vi "GEOM_API.vi"(7 "Cmd":string, 11 "error in":errorcluster) -> (4 "ImmedReplyString":string, 15 "error out":errorcluster)   [LabVIEW 2016]
uses:
  private/vis/GEOM_Coords.ctl
  private/vis/GEOM_VAR_action.ctl
  DBSHAND/private/vis/DatabaseHand_Element_Set(bool).vi
  DBSHAND/private/vis/DatabaseHand_Element_Set(string).vi
  DBSHAND/private/vis/DatabaseHand_Element_Get(bool).vi
panel:
  in  "optimize":bool=TRUE
  in  "overwcs":path
  in  "hdrmoddir":path
  out "header template":path
  out "ConfigFile":path
  in  "bin_correction_type":string="add2pre"
  out "FPA":string
  in  "correction_type":string="simetrical_used_columns"
  in  "ConfigVariables":string[][](table)=[["DATABASE", "path", "GEOM_API.vi", "database_path", "/home/ArcVIEW/Modules/GEOM/public/database", "PATH"], ["ROI", "correction", "GEOM_API.vi", "correction_type", "simetrical_used_columns", "STR"], ["BINNING", "correction", "GEOM_API.vi", "bin_correction_type", "add2pre", "STR"], ["HDRINFO", "hdrmoddir", "GEOM_API.vi", "hdrmoddir", "", "PATH"], ["HDRINFO", "overwcs", "GEOM_API.vi", "overwcs", "", "PATH"], ["MISC", "optimize", "GEOM_API.vi", "optimize", "", "BOOL"]]
  out "Initialized":bool
  in  "database_path":path=path "/__none__"
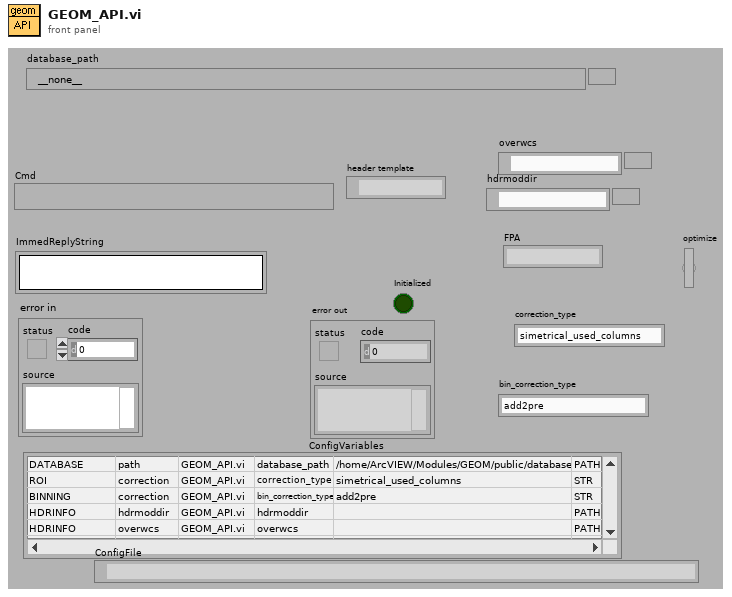
[diagram p1: front panel]
types:
  T1 = typedef "GEOM_VAR_action.ctl" = enum16{"read", "write"}
  T2 = typedef "GEOM_Coords.ctl" = cluster{"xstart":u32, "ystart":u32, "xsize":u32, "ysize":u32}
  T3 = typedef "DatabaseHand_RefNum.ctl" = refnum<vi>
  T4 = typedef "GEOM_HeaderModule.ctl" = cluster{"name":string, "Keys":string[][]}
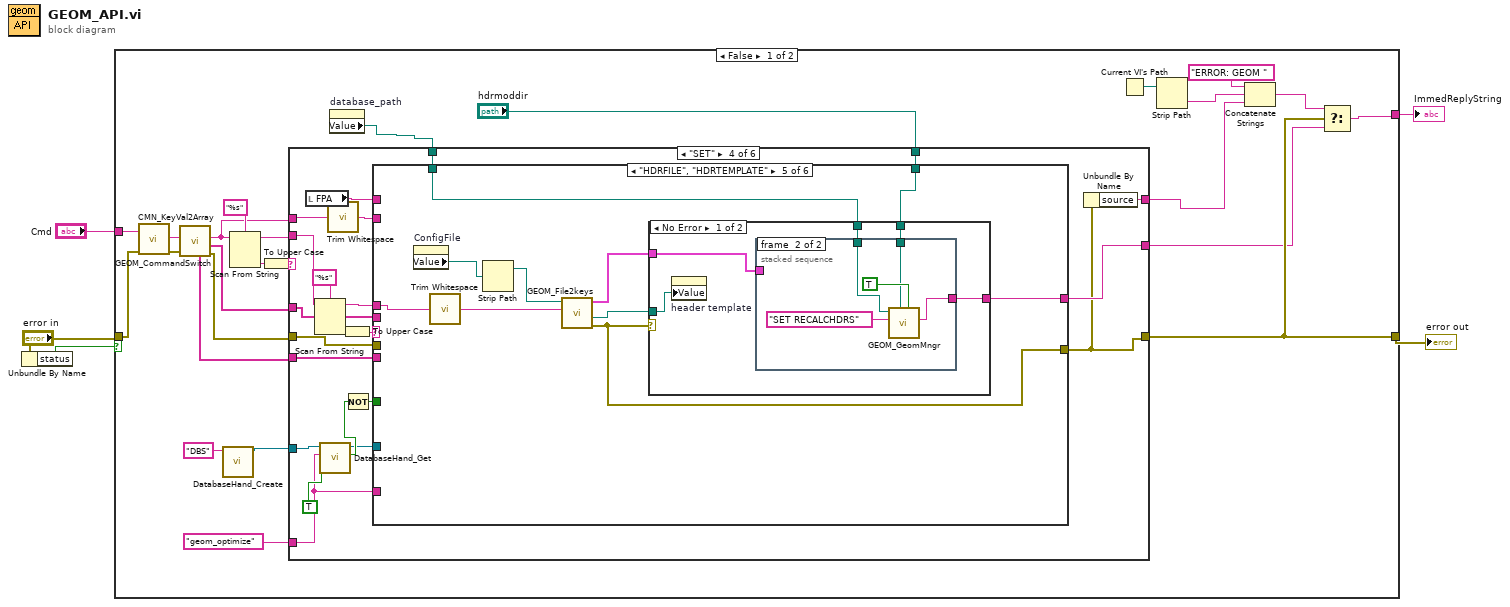
[diagram p0: block diagram]
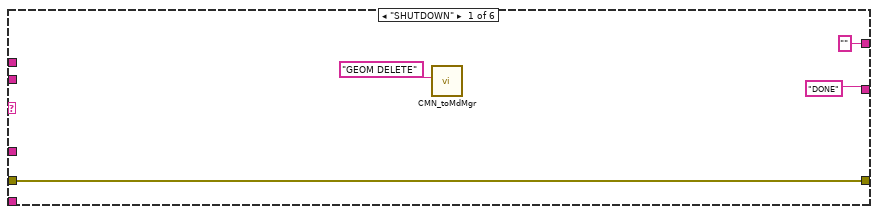
[diagram p2: hidden frame]
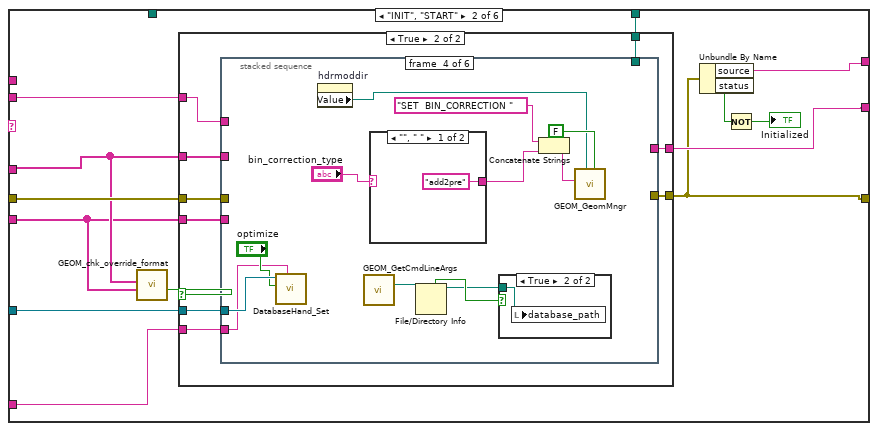
[diagram p3: hidden frame]
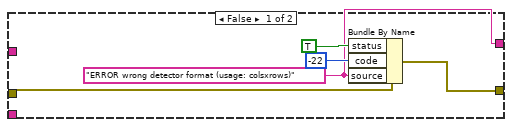
[diagram p4: hidden frame]
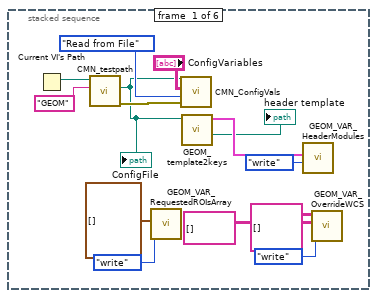
[diagram p5: hidden frame]
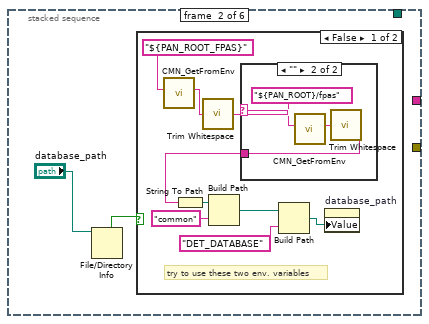
[diagram p6: hidden frame]
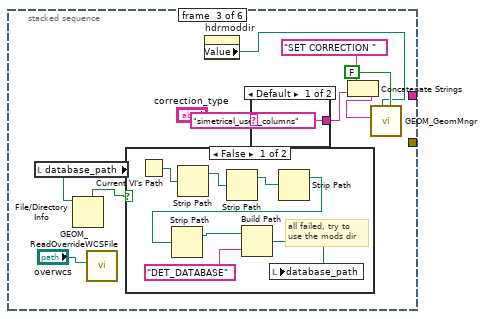
[diagram p9: hidden frame]
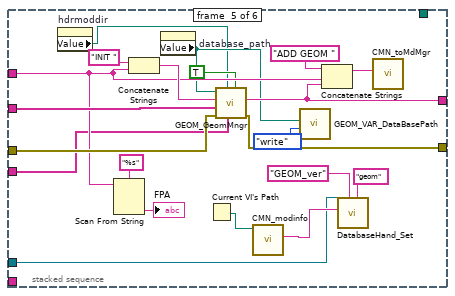
[diagram p14: hidden frame]
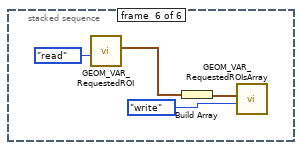
[diagram p15: hidden frame]
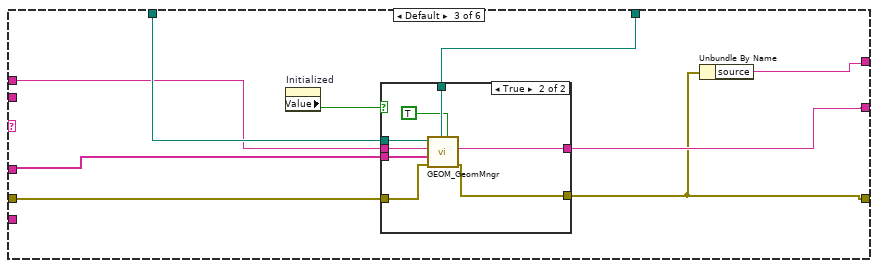
[diagram p16: hidden frame]
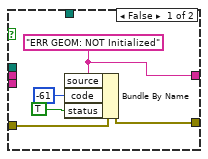
[diagram p17: hidden frame]
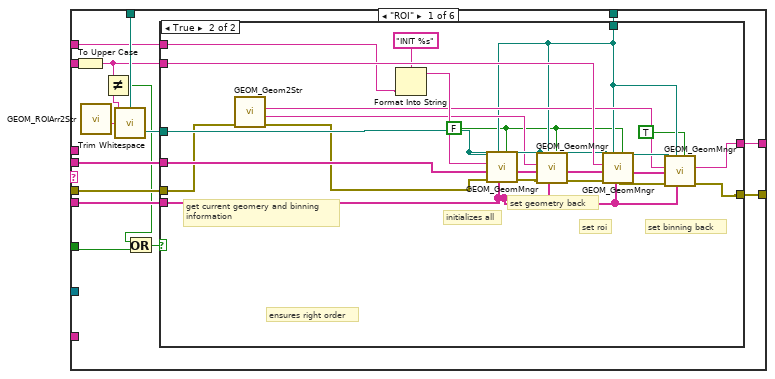
[diagram p18: hidden frame]
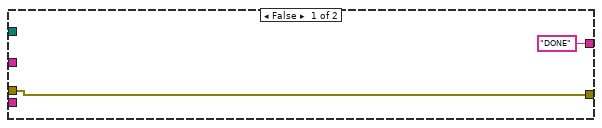
[diagram p19: hidden frame]
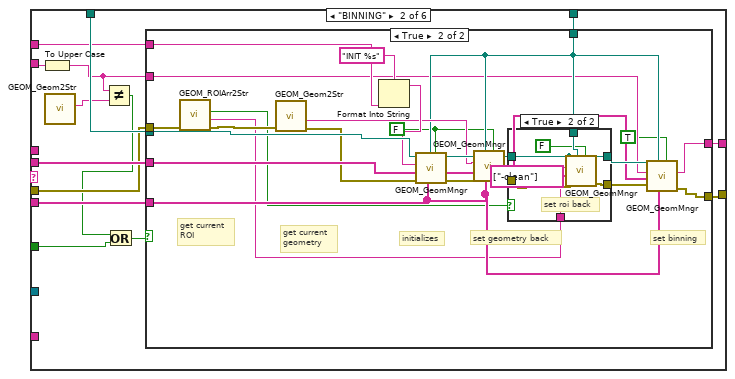
[diagram p20: hidden frame]
diagram:
  n1 = Unbundle By Name("error in") -> ("status"=w3:bool)
  n2 = case shown="False" w3 {
    tunnel: "error in" -> [w17 w457]
    tunnel: [w30 w457] -> w1
    tunnel: [w29 ""] -> w5
    tunnel: "Cmd" -> [w18 _]
    frame False {
      n3 = call "CMN_KeyVal2Array.vi"("error in (no error)"=w17, "command in"=w18) -> ("error out"=w16:errorcluster, "commands out"=w12:string)  [unwired: 1 in, 6 out]
      n4 = call "GEOM_CommandSwitch.vi"("error in (no error)"=w16, "command in"=w12) -> ("error out"=w15:errorcluster, "swhitches"=w13:string[], "command out"=w14:string, "arguments"=w11:string[])  [unwired: 6 out]
      n5 = call "DatabaseHand_Create.vi"("Name"="DBS") -> ("Database RefNum out"=w8:T3)  [unwired: 1 in, 9 out]
      n6 = Scan From String(format string="%s" ("Format String"), input string=w14) -> (remaining string=w20:string, output 1=w28:string)  [unwired: 2 in, 3 out]
      n7 = To Upper Case(1:w28) -> (0:w19:string)
      n8 = property on="database_path" class="Path"() -> ("Value"=w6:path)  [unwired: 2 in, 2 out]
      n9 = case shown="\"SET\"" w19 {
        tunnel: w15 -> [w32 w47 w157 w188 w405 w450]
        tunnel: [w32 w45 w155 w184 w403 w449] -> w30
        tunnel: ["" ("source") w44 w154 w183 w402 w448] -> w22
        tunnel: ["DONE" w46 w156 w185 w404 w448] -> w21
        tunnel: w20 -> [_ w43 _ w192 w398 _]
        tunnel: w14 -> [_ _ w151 w189 w399 _]
        tunnel: w6 -> [_ _ w153 w186 w401 _]
        tunnel: w13 -> [_ w40 w152 w187 w400 w455]
        tunnel: w11 -> [_ w39 _ w181 _ _]
        tunnel: "hdrmoddir" -> [_ w37 w149 w180 w393 _]
        tunnel: w8 -> [_ w36 _ w176 w392 _]
        tunnel: "geom_optimize" ("name") -> [_ w35 _ w171 w391 _]
        frame "SHUTDOWN" {
          n10 = call "CMN_toMdMgr.vi"("command"="GEOM DELETE" ("Command")) -> ()  [unwired: 10 out]
        }
        frame "INIT", "START" {
          n11 = call "GEOM_chk_override_format.vi"("arguments"=w39, "switches"=w40) -> ("format OK"=w38:bool)  [unwired: 9 out]
          n12 = case shown="True" w38 {
            tunnel: w47 -> [w52 w61]
            tunnel: [w48 w60] -> w46
            tunnel: [w49 w59] -> w45
            tunnel: w43 -> [_ w58]
            tunnel: w40 -> [_ w57]
            tunnel: w39 -> [_ w56]
            tunnel: w37 -> [_ w55]
            tunnel: w36 -> [_ w54]
            tunnel: w35 -> [_ w53]
            frame False {
              w48 = "ERROR wrong detector format (usage: colsxrows)" ("source")
              n13 = Bundle By Name(cluster=w52, "status"=TRUE, "code"=-22, "source"=w48) -> (w49:errorcluster)
            }
            frame True {
              n14 = stacked-sequence {
                tunnel: w61 -> [_ _ _ _ w144 _]
                tunnel: [_ _ _ _ w137 _] -> w60
                tunnel: [_ _ _ _ w143 _] -> w59
                tunnel: w58 -> [_ _ _ _ w136 _]
                tunnel: w57 -> [_ _ _ _ w140 _]
                tunnel: w56 -> [_ _ _ _ w129 _]
                tunnel: w55 -> [_ _ _ _ _ _]
                tunnel: w54 -> [_ _ _ w113 w125 _]
                tunnel: w53 -> [_ _ _ w111 _ _]
                frame #0 {
                  n15 = Current VI's Path() -> (path=w75:path)
                  n16 = call "CMN_testpath.vi"("ModuleName"="GEOM", "caller Path"=w75) -> ("error out"=w72:errorcluster, "ConfigFile"=w70:path)  [unwired: 1 in, 7 out]
                  "ConfigFile" <- w70
                  n17 = call "GEOM_VAR_RequestedROIsArray.vi"("Action"=GEOM_VAR_action."write", "ROIs"=T2[] []) -> ()  [unwired: 10 out]
                  n18 = call "CMN_ConfigVals.vi"("error in (no error)"=w72, "Action"=enum16{"Read from File", "Write to File"}."Read from File", "ConfigVariables"="ConfigVariables", "configuration file path"=w70) -> ()  [unwired: 8 out]
                  n19 = call "GEOM_template2keys.vi"("file"=w70) -> ("header template"=→"header template":path, "HeaderModules"=w69:T4[])  [unwired: 1 in, 8 out]
                  n20 = call "GEOM_VAR_HeaderModules.vi"("Action"=GEOM_VAR_action."write", "GEOM_HeaderModules"=w69) -> ()  [unwired: 10 out]
                  n21 = call "GEOM_VAR_OverrideWCS.vi"("Action"=GEOM_VAR_action."write", "override headers"=string[][] [], "override headers mext"=string[][][] []) -> ()  [unwired: 9 out]
                }
                frame #1 {
                  n22 = File/Directory Info(path="database_path") -> (directory=w77:bool)  [unwired: 1 in, 6 out]
                  n23 = case shown="False" w77 {
                    frame False {
                      # "try to use these two env. variables"
                      n24 = call "CMN_GetFromEnv.vi"("str in"="${PAN_ROOT_FPAS}") -> ("str out"=w85:string)  [unwired: 10 out]
                      n25 = call <vilib>:"Trim Whitespace.vi"("string"=w85) -> ("trimmed string"=w84:string)  [unwired: 1 in]
                      n26 = case shown="\"\"" w84 {
                        selector: w84 -> [w87 _]
                        tunnel: [w87 w88] -> w83
                        frame Default {
                        }
                        frame "" {
                          n27 = call "CMN_GetFromEnv.vi"("str in"="${PAN_ROOT}/fpas") -> ("str out"=w89:string)  [unwired: 10 out]
                          n28 = call <vilib>:"Trim Whitespace.vi"("string"=w89) -> ("trimmed string"=w88:string)  [unwired: 1 in]
                        }
                      }
                      n29 = String To Path(string=w83) -> (path=w82:path)
                      n30 = Build Path(base path=w82, name or relative path="common") -> (appended path=w80:path)
                      n31 = Build Path(base path=w80, name or relative path="DET_DATABASE") -> (appended path=w78:path)
                      n32 = property on="database_path" class="Path"("Value"=w78) -> ()  [unwired: 2 in, 2 out]
                    }
                    frame True {
                      # "specified in config file"
                    }
                  }
                }
                frame #2 {
                  n33 = local read "database_path"() -> (w99:path)
                  n34 = File/Directory Info(path=w99) -> (directory=w98:bool)  [unwired: 1 in, 6 out]
                  n35 = call "GEOM_ReadOverrideWCSFile.vi"("Path"="overwcs") -> ()  [unwired: 11 out]
                  n36 = case shown="False" w98 {
                    frame False {
                      # "all failed, try to\nuse the mods dir"
                      n37 = Current VI's Path() -> (path=w108:path)
                      n38 = Strip Path(path=w108) -> (stripped path=w107:path)  [unwired: 1 out]
                      n39 = Strip Path(path=w107) -> (stripped path=w106:path)  [unwired: 1 out]
                      n40 = Strip Path(path=w106) -> (stripped path=w105:path)  [unwired: 1 out]
                      n41 = Strip Path(path=w105) -> (stripped path=w104:path)  [unwired: 1 out]
                      n42 = Build Path(base path=w104, name or relative path="DET_DATABASE") -> (appended path=w102:path)
                      n43 = local write "database_path"(w102) -> ()
                    }
                    frame True {
                    }
                  }
                  n44 = property on="hdrmoddir" class="Path"() -> ("Value"=w91:path)  [unwired: 2 in, 2 out]
                  n45 = case shown="Default" "correction_type" {
                    selector: "correction_type" -> [_ w101]
                    tunnel: ["simetrical_used_columns" w101] -> w95
                    frame Default {
                    }
                    frame "simetrical_all_columns" {
                    }
                  }
                  n46 = Concatenate Strings("SET CORRECTION " ("string"), w95) -> (w94:string)
                  n47 = call "GEOM_GeomMngr.vi"("calc headers?"=FALSE, "hdrmodspath"=w91, "command"=w94) -> ()  [unwired: 4 in, 5 out]
                }
                frame #3 {
                  n48 = call-poly "DatabaseHand_Set.vi"("name"=w111, "value"="optimize", "Database RefNum in"=w113) -> ()  [unwired: 5 in, 4 out]
                  n49 = property on="hdrmoddir" class="Path"() -> ("Value"=w109:path)  [unwired: 2 in, 2 out]
                  n50 = call "GEOM_GetCmdLineArgs.vi"() -> ("det_database"=w116:path)  [unwired: 15 out]
                  n51 = case shown="\"\", \" \"" "bin_correction_type" {
                    selector: "bin_correction_type" -> [_ w123]
                    tunnel: ["add2pre" w123] -> w117
                    frame "", " " {
                    }
                    frame Default {
                    }
                  }
                  n52 = File/Directory Info(path=w116) -> (path out=w114:path, directory=w115:bool)  [unwired: 1 in, 5 out]
                  n53 = case shown="True" w115 {
                    tunnel: w114 -> [_ w121]
                    frame False {
                    }
                    frame True {
                      n54 = local write "database_path"(w121) -> ()
                    }
                  }
                  n55 = Concatenate Strings("SET  BIN_CORRECTION " ("string"), w117) -> (w118:string)
                  n56 = call "GEOM_GeomMngr.vi"("calc headers?"=FALSE, "hdrmodspath"=w109, "command"=w118) -> ()  [unwired: 4 in, 5 out]
                }
                frame #4 {
                  n57 = property on="hdrmoddir" class="Path"() -> ("Value"=w124:path)  [unwired: 2 in, 2 out]
                  n58 = Scan From String(format string="%s", input string=w136) -> (output 1=→"FPA":string)  [unwired: 2 in, 4 out]
                  n59 = Concatenate Strings("INIT ", w136) -> (w141:string)
                  n60 = property on="database_path" class="Path"() -> ("Value"=w127:path)  [unwired: 2 in, 2 out]
                  n61 = Current VI's Path() -> (path=w133:path)
                  n62 = call "GEOM_GeomMngr.vi"("calc headers?"=TRUE, "arguments"=w129, "hdrmodspath"=w124, "error in (no error)"=w144, "switches"=w140, "command"=w141, "database path"=w127) -> ("error out"=w143:errorcluster, "response"=w137:string)  [unwired: 3 out]
                  n63 = call "CMN_modinfo.vi"("caller path"=w133) -> ("INFO"=w132:string)  [unwired: 2 in, 8 out]
                  n64 = call "GEOM_VAR_DataBasePath.vi"("Action"=GEOM_VAR_action."write", "Path"=w127) -> ()  [unwired: 10 out]
                  n65 = Concatenate Strings("ADD GEOM " ("command"), w136, w137) -> (w138:string)
                  n66 = call-poly "DatabaseHand_Set.vi"("group"="geom", "name"="GEOM_ver", "value"=w132, "Database RefNum in"=w125) -> ()  [unwired: 4 in, 4 out]
                  n67 = call "CMN_toMdMgr.vi"("command"=w138) -> ()  [unwired: 10 out]
                }
                frame #5 {
                  n68 = call "GEOM_VAR_RequestedROI.vi"("Action"=GEOM_VAR_action."read") -> ("GEOM_RequestedROI out"=w145:T2)  [unwired: 1 in, 9 out]
                  n69 = Build Array(w145) -> (w147:T2[])
                  n70 = call "GEOM_VAR_RequestedROIsArray.vi"("Action"=GEOM_VAR_action."write", "ROIs"=w147) -> ()  [unwired: 10 out]
                }
              }
            }
          }
          n71 = Unbundle By Name(w45) -> ("source"=w44:string, "status"=w42:bool)
          n72 = Not(x=w42) -> (.not. x?=→"Initialized":bool)
        }
        frame Default {
          n73 = property on="Initialized" class="Bool (strict)"() -> ("Value"=w150:bool)  [unwired: 2 in, 2 out]
          n74 = case shown="True" w150 {
            tunnel: w157 -> [w162 w170]
            tunnel: [w159 w169] -> w156
            tunnel: [w161 w168] -> w155
            tunnel: w153 -> [_ w167]
            tunnel: w152 -> [_ w166]
            tunnel: w151 -> [_ w165]
            tunnel: w149 -> [_ w164]
            frame False {
              w159 = "ERR GEOM: NOT Initialized" ("source")
              n75 = Bundle By Name(cluster=w162, "source"=w159, "code"=-61, "status"=TRUE) -> (w161:errorcluster)
            }
            frame True {
              n76 = call "GEOM_GeomMngr.vi"("calc headers?"=TRUE, "hdrmodspath"=w164, "error in (no error)"=w170, "switches"=w166, "command"=w165, "database path"=w167) -> ("error out"=w168:errorcluster, "response"=w169:string)  [unwired: 1 in, 3 out]
            }
          }
          n77 = Unbundle By Name(w155) -> ("source"=w154:string)
        }
        frame "SET" {
          n78 = local read "FPA"() -> (w182:string)
          n79 = Scan From String(format string="%s", input string=w192) -> (remaining string=w177:string, output 1=w191:string)  [unwired: 2 in, 3 out]
          n80 = call-poly "DatabaseHand_Get.vi"("default value"=TRUE, "name"=w171, "Database RefNum in"=w176) -> ("value"=w174:bool, "Database RefNum out"=w172:T3)  [unwired: 2 in, 5 out]
          n81 = call <vilib>:"Trim Whitespace.vi"("string"=w189) -> ("trimmed string"=w179:string)  [unwired: 1 in]
          n82 = To Upper Case(1:w191) -> (0:w178:string)
          n83 = Not(x=w174) -> (.not. x?=w173:bool)
          n84 = case shown="\"HDRFILE\", \"HDRTEMPLATE\"" w178 {
            tunnel: w179 -> [w207 w234 w282 _ _ w375]
            tunnel: w188 -> [w201 w235 w283 _ _ w374]
            tunnel: w187 -> [w202 w238 w285 _ _ w373]
            tunnel: w186 -> [w206 w242 w287 _ w342 w372]
            tunnel: [w205 w241 w290 errorcluster {"status"=FALSE, "code"=0, "source"=""} ("error out") w347 w371] -> w184
            tunnel: [w204 w240 w289 w327 w346 w370] -> w185
            tunnel: w182 -> [w203 w239 w288 _ _ _]
            tunnel: w181 -> [w200 w237 w284 _ _ w369]
            tunnel: w180 -> [w199 w236 w286 _ w343 w368]
            tunnel: w177 -> [_ _ _ w330 w349 _]
            tunnel: w173 -> [w195 w230 w276 _ _ _]
            tunnel: w172 -> [_ _ _ w332 _ _]
            tunnel: w171 -> [_ _ _ w331 _ _]
            frame "ROI" {
              n85 = To Upper Case(1:w207) -> (0:w198:string)
              n86 = call "GEOM_ROIArr2Str.vi"() -> ("ROI command"=w197:string)  [unwired: 1 in, 10 out]
              n87 = call <vilib>:"Trim Whitespace.vi"("string"=w197) -> ("trimmed string"=w196:string)  [unwired: 1 in]
              n88 = Not Equal?(x=w198, y=w196) -> (x != y?=w194:bool)
              n89 = Or(x=w194, y=w195) -> (x .or. y?=w193:bool)
              n90 = case shown="True" w193 {
                tunnel: w198 -> [_ w228]
                tunnel: w206 -> [_ w226]
                tunnel: [w209 w225] -> w205
                tunnel: ["DONE" ("response") w224] -> w204
                tunnel: w203 -> [_ w222]
                tunnel: w202 -> [_ w216]
                tunnel: w201 -> [w209 w215]
                tunnel: w200 -> [_ w213]
                tunnel: w199 -> [_ w212]
                frame False {
                }
                frame True {
                  w211 = FALSE ("calc headers?")
                  # "get current geomery and binning\ninformation"
                  # "ensures right order"
                  # "set binning back"
                  # "set roi"
                  # "set geometry back"
                  # "initializes all"
                  n91 = call "GEOM_Geom2Str.vi"("error in (no error)"=w215) -> ("error out"=w214:errorcluster, "geometry command"=w217:string, "binning command"=w220:string)  [unwired: 8 out]
                  n92 = Format Into String(format string="INIT %s", w222) -> (resulting string=w221:string)  [unwired: 2 in, 1 out]
                  n93 = call "GEOM_GeomMngr.vi"("calc headers?"=w211, "arguments"=w213, "hdrmodspath"=w212, "error in (no error)"=w214, "switches"=w216, "command"=w221, "database path"=w226) -> ("error out"=w219:errorcluster)  [unwired: 4 out]
                  n94 = call "GEOM_GeomMngr.vi"("calc headers?"=w211, "arguments"=w213, "hdrmodspath"=w212, "error in (no error)"=w219, "switches"=w216, "command"=w217, "database path"=w226) -> ("error out"=w218:errorcluster)  [unwired: 4 out]
                  n95 = call "GEOM_GeomMngr.vi"("calc headers?"=w211, "arguments"=w213, "hdrmodspath"=w212, "error in (no error)"=w218, "switches"=w216, "command"=w228, "database path"=w226) -> ("error out"=w227:errorcluster)  [unwired: 4 out]
                  n96 = call "GEOM_GeomMngr.vi"("calc headers?"=TRUE, "arguments"=w213, "hdrmodspath"=w212, "error in (no error)"=w227, "switches"=w216, "command"=w220, "database path"=w226) -> ("error out"=w225:errorcluster, "response"=w224:string)  [unwired: 3 out]
                }
              }
            }
            frame "BINNING" {
              n97 = To Upper Case(1:w234) -> (0:w233:string)
              n98 = call "GEOM_Geom2Str.vi"() -> ("binning command"=w232:string)  [unwired: 1 in, 10 out]
              n99 = Not Equal?(x=w233, y=w232) -> (x != y?=w231:bool)
              n100 = Or(x=w231, y=w230) -> (x .or. y?=w229:bool)
              n101 = case shown="True" w229 {
                tunnel: w242 -> [_ w266]
                tunnel: [w244 w262] -> w241
                tunnel: ["DONE" ("response") w260] -> w240
                tunnel: w239 -> [_ w259]
                tunnel: w238 -> [_ w257]
                tunnel: w237 -> [_ w253]
                tunnel: w236 -> [_ w252]
                tunnel: w235 -> [w244 w251]
                tunnel: w233 -> [_ w247]
                frame False {
                  # "nothing to do"
                }
                frame True {
                  w246 = FALSE ("calc headers?")
                  # "set binning"
                  # "set geometry back"
                  # "initializes"
                  # "get current \ngeometry"
                  # "get current \nROI"
                  n102 = call "GEOM_ROIArr2Str.vi"("error in (no error)"=w251) -> ("error out"=w250:errorcluster, "ROI command"=w248:string, "defined?"=w249:bool)  [unwired: 8 out]
                  n103 = call "GEOM_Geom2Str.vi"("error in (no error)"=w250) -> ("error out"=w254:errorcluster, "geometry command"=w255:string)  [unwired: 9 out]
                  n104 = Format Into String(format string="INIT %s", w259) -> (resulting string=w264:string)  [unwired: 2 in, 1 out]
                  n105 = call "GEOM_GeomMngr.vi"("calc headers?"=w246, "arguments"=w253, "hdrmodspath"=w252, "error in (no error)"=w254, "switches"=w257, "command"=w264, "database path"=w266) -> ("error out"=w258:errorcluster)  [unwired: 4 out]
                  n106 = call "GEOM_GeomMngr.vi"("calc headers?"=w246, "arguments"=w253, "hdrmodspath"=w252, "error in (no error)"=w258, "switches"=w257, "command"=w255, "database path"=w266) -> ("error out"=w256:errorcluster)  [unwired: 4 out]
                  n107 = case shown="True" w249 {
                    tunnel: w266 -> [w268 w273]
                    tunnel: [w267 w275] -> w263
                    tunnel: w256 -> [w267 w274]
                    tunnel: [w268 w273] -> w261
                    tunnel: w248 -> [_ w271]
                    tunnel: w252 -> [_ w270]
                    frame False {
                      # "no roi efined"
                    }
                    frame True {
                      # "set roi back"
                      n108 = call "GEOM_GeomMngr.vi"("calc headers?"=FALSE, "hdrmodspath"=w270, "error in (no error)"=w274, "switches"=string[] ["-clean"], "command"=w271, "database path"=w273) -> ("error out"=w275:errorcluster)  [unwired: 1 in, 4 out]
                    }
                  }
                  n109 = call "GEOM_GeomMngr.vi"("calc headers?"=TRUE, "arguments"=w253, "hdrmodspath"=w252, "error in (no error)"=w263, "switches"=w257, "command"=w247, "database path"=w261) -> ("error out"=w262:errorcluster, "response"=w260:string)  [unwired: 3 out]
                }
              }
            }
            frame "GEOMETRY" {
              n110 = To Upper Case(1:w282) -> (0:w280:string)
              n111 = call "GEOM_Geom2Str.vi"() -> ("geometry command"=w281:string)  [unwired: 1 in, 10 out]
              n112 = call <vilib>:"Trim Whitespace.vi"("string"=w281) -> ("trimmed string"=w279:string)  [unwired: 1 in]
              n113 = Not Equal?(x=w280, y=w279) -> (x != y?=w278:bool)
              n114 = Or(x=w278, y=w276) -> (x .or. y?=w277:bool)
              n115 = case shown="True" w277 {
                tunnel: [w292 w313] -> w290
                tunnel: ["DONE" ("response") w311] -> w289
                tunnel: w288 -> [_ w310]
                tunnel: w280 -> [_ w306]
                tunnel: w287 -> [_ w305]
                tunnel: w286 -> [_ w303]
                tunnel: w285 -> [_ w296]
                tunnel: w284 -> [_ w295]
                tunnel: w283 -> [w292 w300]
                frame False {
                }
                frame True {
                  w293 = FALSE ("calc headers?")
                  # "set orig geometry"
                  # "set binning back"
                  # "set new geometry"
                  # "initializes"
                  # "get current \nbinning"
                  # "get current \nROI"
                  n116 = call "GEOM_ROIArr2Str.vi"("error in (no error)"=w300) -> ("error out"=w298:errorcluster, "ROI command"=w297:string, "defined?"=w299:bool)  [unwired: 8 out]
                  n117 = call "GEOM_Geom2Str.vi"("error in (no error)"=w298) -> ("error out"=w308:errorcluster, "geometry command"=w302:string, "binning command"=w307:string)  [unwired: 8 out]
                  n118 = Format Into String(format string="INIT %s", w310) -> (resulting string=w315:string)  [unwired: 2 in, 1 out]
                  n119 = call "GEOM_GeomMngr.vi"("calc headers?"=w293, "arguments"=w295, "hdrmodspath"=w303, "error in (no error)"=w308, "switches"=w296, "command"=w315, "database path"=w305) -> ("error out"=w304:errorcluster)  [unwired: 4 out]
                  n120 = call "GEOM_GeomMngr.vi"("calc headers?"=w293, "hdrmodspath"=w303, "error in (no error)"=w304, "switches"=w296, "command"=w302, "database path"=w305) -> ("error out"=w301:errorcluster)  [unwired: 1 in, 4 out]
                  n121 = call "GEOM_GeomMngr.vi"("calc headers?"=w293, "arguments"=w295, "hdrmodspath"=w303, "error in (no error)"=w301, "switches"=w296, "command"=w306, "database path"=w305) -> ("error out"=w309:errorcluster)  [unwired: 4 out]
                  n122 = case shown="True" w299 {
                    tunnel: w305 -> [w318 w323]
                    tunnel: [w317 w325] -> w314
                    tunnel: w309 -> [w317 w324]
                    tunnel: [w318 w323] -> w312
                    tunnel: w297 -> [_ w322]
                    tunnel: w303 -> [_ w321]
                    tunnel: w296 -> [_ _]
                    frame False {
                      # "no roi efined"
                    }
                    frame True {
                      # "set roi back"
                      n123 = call "GEOM_GeomMngr.vi"("calc headers?"=FALSE, "hdrmodspath"=w321, "error in (no error)"=w324, "switches"=string[] ["-clean"], "command"=w322, "database path"=w323) -> ("error out"=w325:errorcluster)  [unwired: 1 in, 4 out]
                    }
                  }
                  n124 = call "GEOM_GeomMngr.vi"("calc headers?"=TRUE, "arguments"=w295, "hdrmodspath"=w303, "error in (no error)"=w314, "switches"=w296, "command"=w307, "database path"=w312) -> ("error out"=w313:errorcluster, "response"=w311:string)  [unwired: 3 out]
                }
              }
            }
            frame "GEOM_OPTIMIZE", "OPTIMIZE" {
              n125 = Scan From String(format string="%s", input string=w330) -> (output 1=w328:string)  [unwired: 2 in, 4 out]
              n126 = case shown="Default" w328 {
                tunnel: w332 -> [_ w337 w341]
                tunnel: w331 -> [_ w336 w340]
                tunnel: ["ERROR <on | off>" ("response") "DONE" ("response") "DONE" ("response")] -> w327
                frame Default {
                }
                frame "1", "on", "true", "yes" {
                  n127 = call-poly "DatabaseHand_Set.vi"("name"=w336, "value"=TRUE, "Database RefNum in"=w337) -> ()  [unwired: 5 in, 4 out]
                }
                frame "0", "false", "no", "off" {
                  n128 = call-poly "DatabaseHand_Set.vi"("name"=w340, "value"=FALSE, "Database RefNum in"=w341) -> ()  [unwired: 5 in, 4 out]
                }
              }
            }
            frame "HDRFILE", "HDRTEMPLATE" {
              n129 = property on="ConfigFile" class="Path"() -> ("Value"=w351:path)  [unwired: 2 in, 2 out]
              n130 = call <vilib>:"Trim Whitespace.vi"("string"=w349) -> ("trimmed string"=w348:string)  [unwired: 1 in]
              n131 = Strip Path(path=w351) -> (stripped path=w350:path)  [unwired: 1 out]
              n132 = call "GEOM_File2keys.vi"("template in"=w348, "ref dir"=w350) -> ("error out"=w347:errorcluster, "header template"=w345:path, "HeaderModules"=w344:T4[])  [unwired: 1 in, 6 out]
              n133 = case shown="No Error" w347 {
                selector: w347 -> [_ w367]
                tunnel: [w355 w364] -> w346
                tunnel: w345 -> [w354 _]
                tunnel: w344 -> [w356 _]
                tunnel: w343 -> [w353 _]
                tunnel: w342 -> [w352 _]
                frame No Error {
                  n134 = property on="header template" class="Path"("Value"=w354) -> ()  [unwired: 2 in, 2 out]
                  n135 = stacked-sequence {
                    tunnel: w356 -> [w357 _]
                    tunnel: [_ w362] -> w355
                    tunnel: w353 -> [_ w360]
                    tunnel: w352 -> [_ w359]
                    frame #0 {
                      n136 = call "GEOM_VAR_HeaderModules.vi"("Action"=GEOM_VAR_action."write", "GEOM_HeaderModules"=w357) -> ()  [unwired: 10 out]
                    }
                    frame #1 {
                      n137 = call "GEOM_GeomMngr.vi"("calc headers?"=TRUE, "hdrmodspath"=w360, "command"="SET RECALCHDRS", "database path"=w359) -> ("response"=w362:string)  [unwired: 3 in, 4 out]
                    }
                  }
                }
                frame Error {
                  n138 = Unbundle By Name(w367) -> ("code"=w366:i32)
                  n139 = Format Into String(format string="ERROR (%d) reading template", w366) -> (resulting string=w364:string)  [unwired: 2 in, 1 out]
                }
              }
            }
            frame Default {
              n140 = property on="Initialized" class="Bool (strict)"() -> ("Value"=w376:bool)  [unwired: 2 in, 2 out]
              n141 = case shown="True" w376 {
                tunnel: w374 -> [w381 w385]
                tunnel: [w378 w390] -> w370
                tunnel: [w380 w389] -> w371
                tunnel: w372 -> [_ w388]
                tunnel: w373 -> [_ w387]
                tunnel: w375 -> [_ w386]
                tunnel: w369 -> [_ w384]
                tunnel: w368 -> [_ w383]
                frame False {
                  w378 = "ERR GEOM: NOT Initialized" ("source")
                  n142 = Bundle By Name(cluster=w381, "source"=w378, "code"=-61, "status"=TRUE) -> (w380:errorcluster)
                }
                frame True {
                  n143 = call "GEOM_GeomMngr.vi"("calc headers?"=TRUE, "arguments"=w384, "hdrmodspath"=w383, "error in (no error)"=w385, "switches"=w387, "command"=w386, "database path"=w388) -> ("error out"=w389:errorcluster, "response"=w390:string)  [unwired: 3 out]
                }
              }
            }
          }
          n144 = Unbundle By Name(w184) -> ("source"=w183:string)
        }
        frame "GET" {
          n145 = Scan From String(format string="%s", input string=w398) -> (remaining string=w394:string, output 1=w396:string)  [unwired: 2 in, 3 out]
          n146 = To Upper Case(1:w396) -> (0:w395:string)
          n147 = case shown="\"HDRFILE\", \"HDRTEMPLATE\"" w395 {
            tunnel: w405 -> [w408 w411 w414 w417 w422 w440 w447]
            tunnel: [w406 w410 w413 w416 w420 w433 w446] -> w404
            tunnel: [w408 w411 w414 w417 w421 w440 w445] -> w403
            tunnel: w401 -> [_ _ _ _ w426 _ w444]
            tunnel: w400 -> [_ _ _ _ _ _ w443]
            tunnel: w399 -> [_ _ _ _ _ _ w442]
            tunnel: w394 -> [_ _ _ _ _ _ _]
            tunnel: w393 -> [_ _ _ _ _ _ w441]
            tunnel: w392 -> [_ _ _ _ _ w439 _]
            tunnel: w391 -> [_ _ _ _ _ w438 _]
            frame "DATAPATH" {
              n148 = property on="database_path" class="Path"() -> ("Value"=w407:path)  [unwired: 2 in, 2 out]
              n149 = Path To String(path=w407) -> (string=w406:string)
            }
            frame "CONFIGFILE" {
              n150 = property on="ConfigFile" class="Path"() -> ("Value"=w409:path)  [unwired: 2 in, 2 out]
              n151 = Path To String(path=w409) -> (string=w410:string)
            }
            frame "HDRFILE", "HDRTEMPLATE" {
              n152 = property on="header template" class="Path"() -> ("Value"=w412:path)  [unwired: 2 in, 2 out]
              n153 = Path To String(path=w412) -> (string=w413:string)
            }
            frame "HDRMODDIR", "HDRMODPATH" {
              n154 = property on="hdrmoddir" class="Path"() -> ("Value"=w415:path)  [unwired: 2 in, 2 out]
              n155 = Path To String(path=w415) -> (string=w416:string)
            }
            frame "FPAS" {
              n156 = Build Path(base path=w426, name or relative path="FPA") -> (appended path=w424:path)
              n157 = List Folder(path=w424, pattern="*.fpa", error in=w422) -> (filenames=w423:string[], error out=w421:errorcluster)  [unwired: 3 out]
              n158 = for {
                tunnel: w423 -> [w432] mode=indexing
                shift-right: [w429] -> w420
                shift-left: "" -> [w428]
                n159 = Match Pattern(string=w432, regular expression=".fpa") -> (before substring=w430:string)  [unwired: 4 out]
                n160 = Concatenate Strings(w428, w430, "\n") -> (w429:string)
              }
            }
            frame "GEOM_OPTIMIZE", "OPTIMIZE" {
              n161 = call-poly "DatabaseHand_Get.vi"("default value"=TRUE, "name"=w438, "Database RefNum in"=w439) -> ("value"=w436:bool)  [unwired: 2 in, 6 out]
              n162 = Select(t="on" ("response"), s=w436, f="off") -> (s? t:f=w433:string)
            }
            frame Default {
              n163 = call "GEOM_GeomMngr.vi"("hdrmodspath"=w441, "error in (no error)"=w447, "switches"=w443, "command"=w442, "database path"=w444) -> ("error out"=w445:errorcluster, "response"=w446:string)  [unwired: 2 in, 3 out]
            }
          }
          n164 = Unbundle By Name(w403) -> ("source"=w402:string)
        }
        frame "VERSION" {
          n165 = Search 1D Array(1D array=w455, element="-full") -> (index of element=w453:i32)  [unwired: 1 out]
          n166 = Greater Or Equal To 0?(x=w453) -> (x >= 0?=w452:bool)
          n167 = Current VI's Path() -> (path=w451:path)
          n168 = call "CMN_modinfo.vi"("error in (no error)"=w450, "full"=w452, "caller path"=w451) -> ("error out"=w449:errorcluster, "INFO"=w448:string)  [unwired: 7 out]
        }
      }
      n169 = Current VI's Path() -> (path=w25:path)
      n170 = Strip Path(path=w25) -> (name=w24:string)  [unwired: 1 out]
      n171 = Concatenate Strings("ERROR: GEOM ", w24, w22) -> (w23:string)
      n172 = Select(t=w23, s=w30, f=w21) -> (s? t:f=w29:string)
    }
    frame True {
    }
  }
  "error out" <- w1
  "ImmedReplyString" <- w5
